vi "AlliGator Get Selected, INT & G2 Channel Names.vi"(11 "Selected Channel Name in":string) -> (0 "Dataset Channel":T1, 1 "INT Channel Name (or empty)":string, 3 "G2 Channel Name (or single Channel Name)":string)   [LabVIEW 2021, in "AlliGator Dual-Channel Datasets.lvlib"]
doc: "Formats dual-gate channel name and returns selected channel."
uses:
  AlliGator Dual-Channel Datasets.lvlib
  AlliGator Dataset Channel.ctl
panel:
  # "see the AlliGator License on the block diagram (Ctrl+E or Window:Show Block Diagram)"
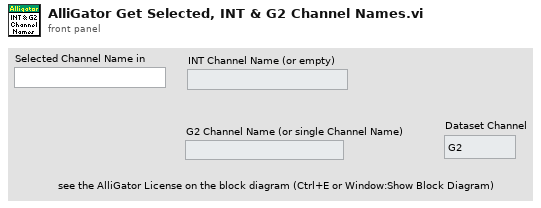
[diagram p1: front panel]
types:
  T1 = typedef "AlliGator Dual-Channel Datasets.lvlib/AlliGator Dataset Channel.ctl" = enum16{"G2", "INT"}
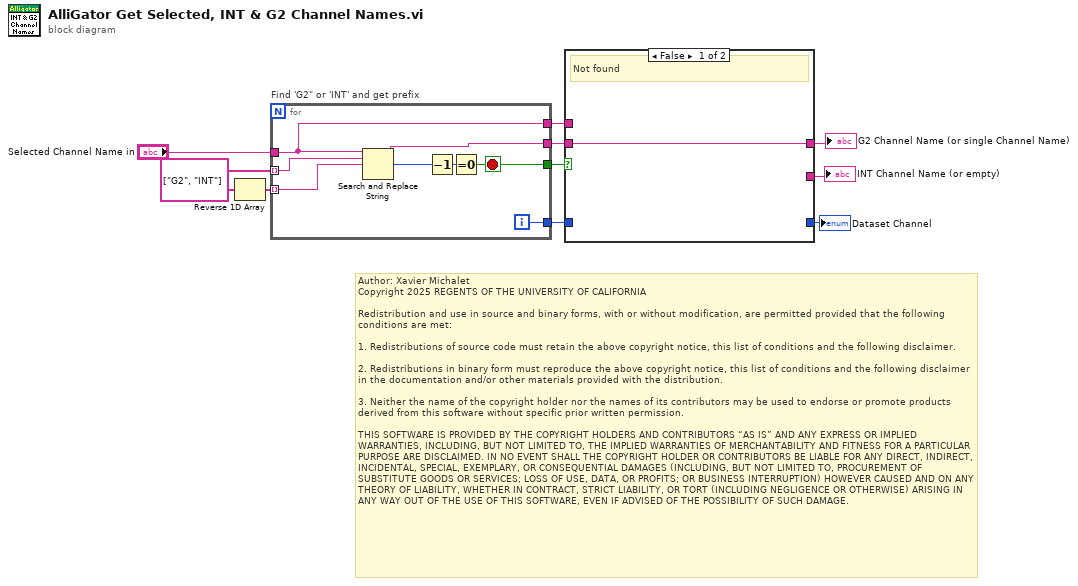
[diagram p0: block diagram]
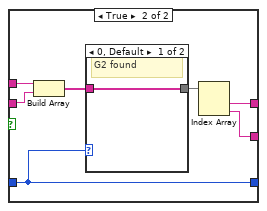
[diagram p2: hidden frame]
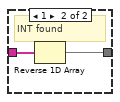
[diagram p3: hidden frame]
diagram:
  w3 = string[] ["G2", "INT"] ("regular expression")
  # "Author: Xavier Michalet\nCopyright 2025 REGENTS OF THE UNIVERSITY OF CALIFORNIA\n\nRedistribution and use in source and binary forms, with or without modification, are permitted provided that the following conditions are met:\n\n1. Redistributions of source code must retain the above copyright notice, this list of conditions and the following disclaimer.\n\n2. Redistributions in binary form must reproduce the above copyright notice, this list of conditions and the following disclaimer in the documentation and/or other materials provided with the distribution.\n\n3. Neither the name of the copyright holder nor the names of its contributors may be used to endorse or promote products derived from this software without specific prior written permission.\n\nTHIS SOFTWARE IS PROVIDED BY THE COPYRIGHT HOLDERS AND CONTRIBUTORS “AS IS” AND ANY EXPRESS OR IMPLIED WARRANTIES, INCLUDING, BUT NOT LIMITED TO, THE IMPLIED WARRANTIES OF MERCHANTABILITY AND FITNESS FOR A PARTICULAR PURPOSE ARE DISCLAIMED. IN NO EVENT SHALL THE COPYRIGHT HOLDER OR CONTRIBUTORS BE LIABLE FOR ANY DIRECT, INDIRECT, INCIDENTAL, SPECIAL, EXEMPLARY, OR CONSEQUENTIAL DAMAGES (INCLUDING, BUT NOT LIMITED TO, PROCUREMENT OF SUBSTITUTE GOODS OR SERVICES; LOSS OF USE, DATA, OR PROFITS; OR BUSINESS INTERRUPTION) HOWEVER CAUSED AND ON ANY THEORY OF LIABILITY, WHETHER IN CONTRACT, STRICT LIABILITY, OR TORT (INCLUDING NEGLIGENCE OR OTHERWISE) ARISING IN ANY WAY OUT OF THE USE OF THIS SOFTWARE, EVEN IF ADVISED OF THE POSSIBILITY OF SUCH DAMAGE."
  n1 = Reverse 1D Array(array=w3) -> (reversed array=w2:string[])
  n2 = for "Find 'G2\" or 'INT' and get prefix" {
    tunnel: "Selected Channel Name in" -> [w11]
    tunnel: w3 -> [w15] mode=indexing
    tunnel: [w18] -> w8
    tunnel: [w17] -> w7
    tunnel: [w16] -> w5
    tunnel: w2 -> [w12] mode=indexing
    tunnel: [w11] -> w1
    i -> [w16]
    stop <- w17 stop-if-true
    n3 = Search and Replace String(input string=w11, search string=w15, replace string=w12) -> (result string=w18:string, number of replacements=w14:i32)  [unwired: 5 in, 2 out]
    n4 = Decrement(x=w14) -> (x-1=w13:i32)
    n5 = Equal To 0?(x=w13) -> (x = 0?=w17:bool)
  }
  n6 = case shown="False" w7 {
    tunnel: w8 -> [w19 w24]
    tunnel: [w19 w21] -> w9
    tunnel: [_ w20] -> w10
    tunnel: [_ w26] -> w4
    tunnel: w5 -> [_ w26]
    tunnel: w1 -> [_ w25]
    frame False {
      # "Not found"
    }
    frame True {
      n7 = Build Array(w25, w24) -> (w23:string[])
      n8 = case shown="0, Default" w26 {
        tunnel: w23 -> [w27 w29]
        tunnel: [w27 w28] -> w22
        frame 0, Default {
          # "G2 found"
        }
        frame 1 {
          # "INT found"
          n9 = Reverse 1D Array(array=w29) -> (reversed array=w28:string[])
        }
      }
      n10 = Index Array(array=w22) -> (element #1=w21:string, element #2=w20:string)  [unwired: 2 in]
    }
  }
  "INT Channel Name (or empty)" <- w10
  "G2 Channel Name (or single Channel Name)" <- w9
  "Dataset Channel" <- w4
